vi "Write Encoder.vi"(10 "Encoder":i32, 11 "ValveModbus in":refnum<class "ValveModbus.lvclass">) -> (3 "ValveModbus out":refnum<class "ValveModbus.lvclass">)   [LabVIEW 2019, in "ValveModbus.lvclass"]
uses:
  ValveModbus.lvclass
  ValveModbus.lvclass/ValveModbus.ctl
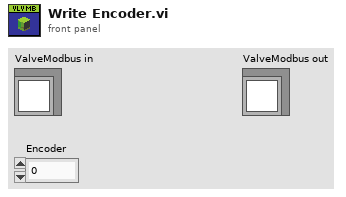
[diagram p1: front panel]
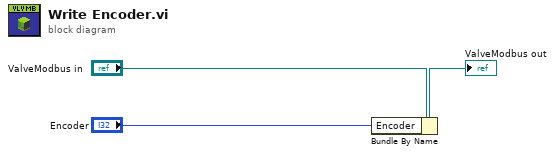
[diagram p0: block diagram]
diagram:
  n1 = Bundle By Name(cluster="ValveModbus in", "Encoder"="Encoder") -> (→"ValveModbus out":refnum<class "ValveModbus.lvclass">)
